vi "SSA.vi"(0 "System no.":i32=1 min=1 max=4 step=1, 2 "Channels to set":string[](array[string]), 3 "Step voltage":dbl[](array[numeric]) format="%.6f", 4 "No.of digits":i16=4, 5 "error in":errorcluster) -> (14 "Controller error":bool, 19 "error out":errorcluster)   [LabVIEW 2020]
doc: "Sets driving voltage amplitude for all kind of step motion of specified PiezoWalk channels. No. of digits is the number of digits after the decimal point in the Step voltage value(s) that will be sent. Hidden error is TRUE if selected system reports error code unequal to 0. \n\nE-755: After changing the step voltage, APG.vi must be run again.\n\nE-861: SSA changes the value of the Bending Voltage parameter (ID 0x07000003) in volatile memory (can be saved as power-on default with WPA, can also be changed with SPA and SEP). \nThe SSA setting takes effect for stepping motion in open-loop operation (servo off). Decreasing the step size will decrease the velocity for open-loop stepping motion. The velocity for open-loop stepping motion is also influenced by the open-loop velocity set with OVL."
panel:
  # "Sets driving voltage amplitude for all kind of step motion of \nspecified PiezoWalk channels."
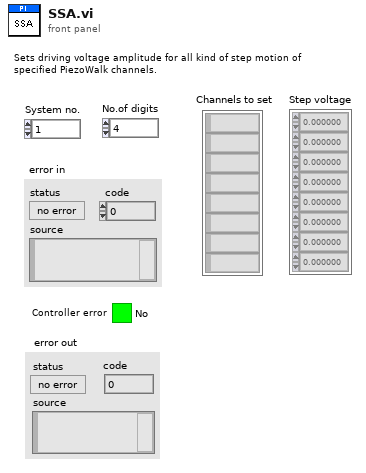
[diagram p1: front panel]
types:
  T1 = enum16{"Disable error check", "Force error check", "Use global settings"}
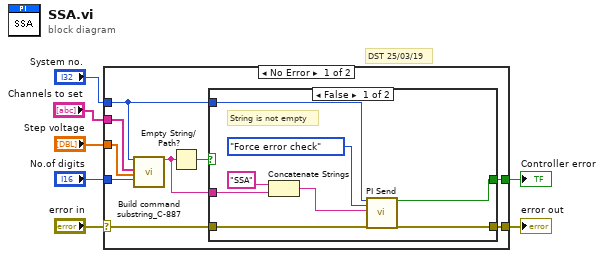
[diagram p0: block diagram]
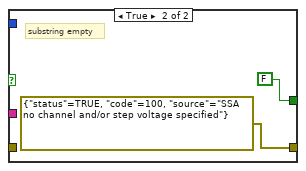
[diagram p2: hidden frame]
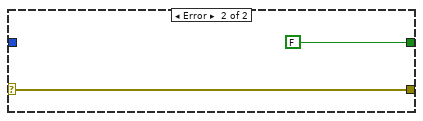
[diagram p3: hidden frame]
diagram:
  # "DST 25/03/19"
  n1 = case shown="No Error" "error in" {
    selector: "error in" -> [w11 w28]
    tunnel: [w16 w28] -> w7
    tunnel: "Step voltage" -> [w15 _]
    tunnel: "No.of digits" -> [w14 _]
    tunnel: "System no." -> [w12 _]
    tunnel: "Channels to set" -> [w13 _]
    tunnel: [w8 FALSE ("Controller error")] -> w1
    frame No Error {
      n2 = call "Build command substring_C-887.vi"("System no."=w12, "Affected axes"=w13, "Parameters"=w15, "No. of digits"=w14) -> ("Command substring"=w10:string)  [unwired: 3 in, 12 out]
      n3 = Empty String/Path?(string/path=w10) -> (empty?=w9:bool)
      n4 = case shown="False" w9 {
        tunnel: w10 -> [w23 _]
        tunnel: [w19 errorcluster {"status"=TRUE, "code"=100, "source"="SSA no channel and/or step voltage specified"} ("error out")] -> w16
        tunnel: w11 -> [w21 _]
        tunnel: w12 -> [w20 _]
        tunnel: [w18 FALSE ("Controller error")] -> w8
        frame False {
          # "String is not empty"
          n5 = Concatenate Strings("SSA", w23) -> (w22:string)
          n6 = call "PI Send.vi"("System no."=w20, "Error check settings"=T1."Force error check", "String to send"=w22, "error in"=w21) -> ("Controller error"=w18:bool, "error out"=w19:errorcluster)  [unwired: 2 in, 12 out]
        }
        frame True {
          # "substring empty"
        }
      }
    }
    frame Error {
    }
  }
  "error out" <- w7
  "Controller error" <- w1
